vi "DoNewModule.vi"(8 "error in (no error)":errorcluster, 9 "ModuleParams":T1, 10 "Save Folder":path, 11 "Project in":refnum<vi>) -> (0 "error out":errorcluster, 3 "Project out":refnum<vi>)   [LabVIEW 2024, in "AddNewModule.lvlib"]
uses:
  AddNewModule.lvlib
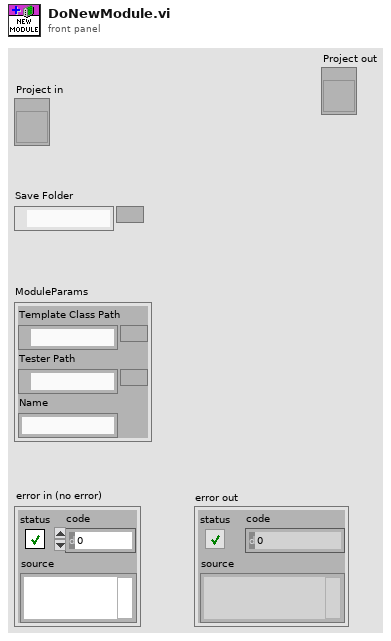
[diagram p1: front panel]
types:
  T1 = cluster{"Template Class Path":path, "Tester Path":path, "Name":string}
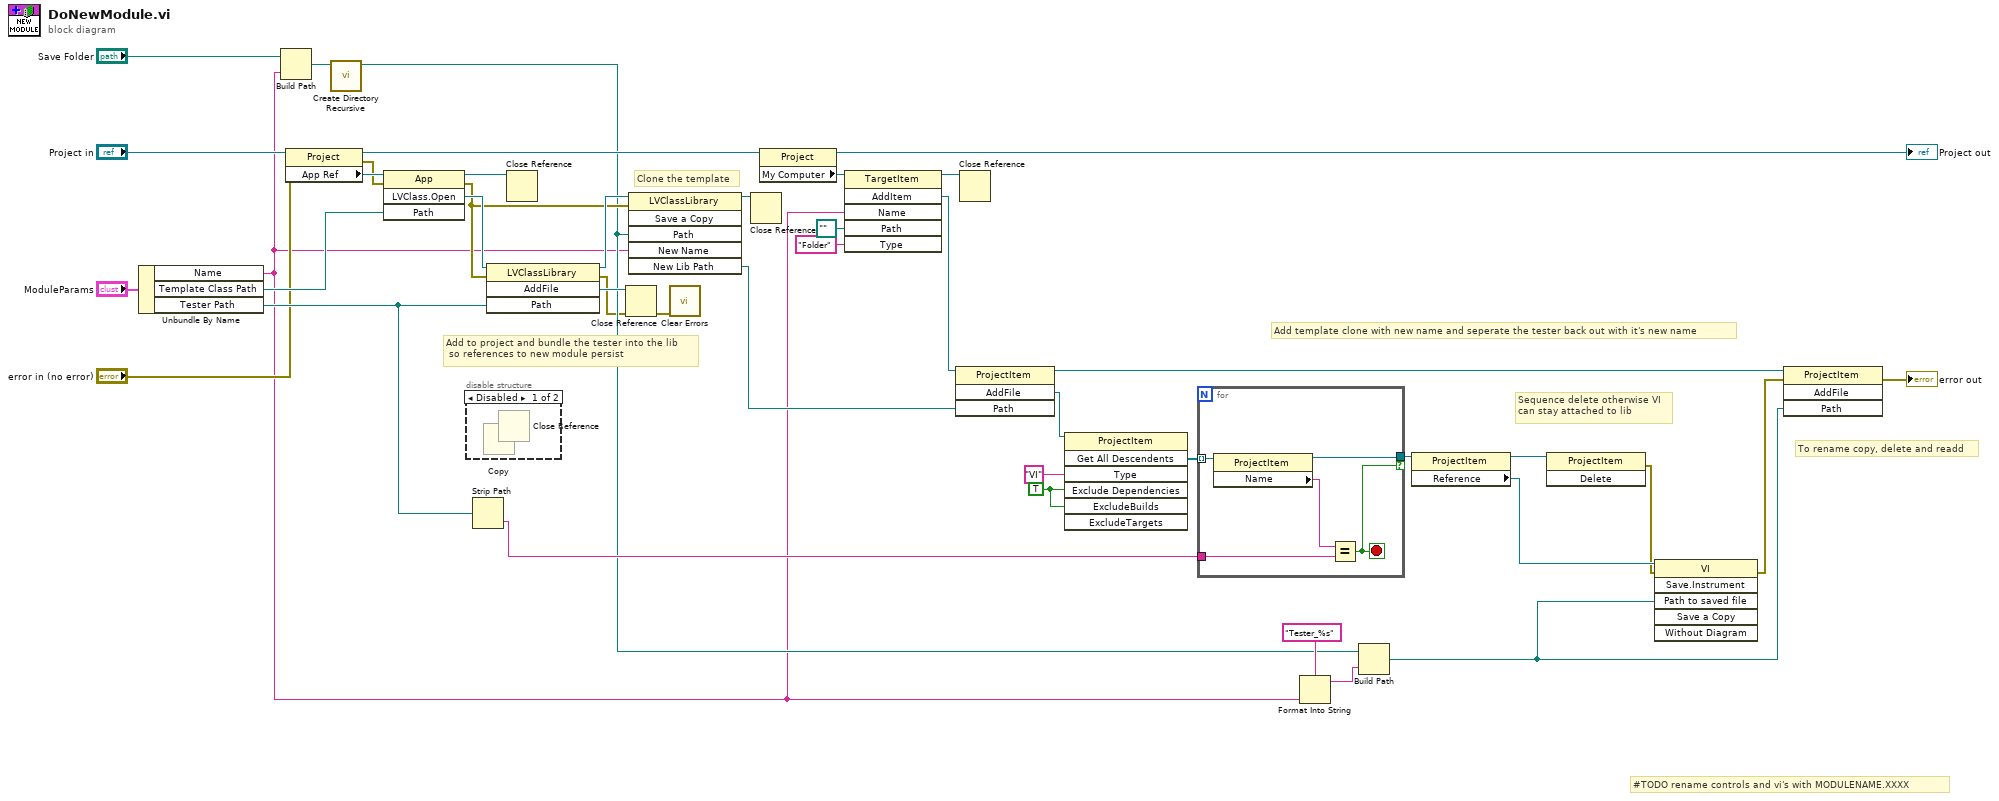
[diagram p0: block diagram]
diagram:
  w21 = TRUE ("ExcludeDependencies")
  # "#TODO rename controls and vi's with MODULENAME.XXXX"
  # "Add template clone with new name and seperate the tester back out with it's new name"
  # "Clone the template"
  # "Add to project and bundle the tester into the lib\n so references to new module persist"
  # "Sequence delete otherwise VI\ncan stay attached to lib"
  # "To rename copy, delete and readd"
  n1 = Unbundle By Name("ModuleParams") -> ("Name"=w1:string, "Template Class Path"=w37:path, "Tester Path"=w24:path)
  n2 = Build Path(base path="Save Folder", name or relative path=w1) -> (appended path=w40:path)
  n3 = property class="Project"(reference="Project in", error in="error in (no error)") -> (reference out=w34:refnum<vi>, error out=w2:errorcluster, "App Ref"=w38:refnum<vi>)
  n4 = call <vilib>:"Create Directory Recursive.vi"("directory"=w40) -> ("directory copy"=w9:path)  [unwired: 4 in, 2 out]
  n5 = invoke class="App" method="LVClass.Open"(reference=w38, error in=w2, "Path"=w37) -> (reference out=w33:refnum<vi>, error out=w30:errorcluster, "LVClass.Open"=w36:refnum<vi>)  [unwired: 1 in, 1 out]
  n6 = disable-structure shown="Disabled" {
    frame Disabled {
      n7 = Copy() -> ()  [unwired: 5 in, 3 out]
      n8 = Close Reference() -> ()  [unwired: 2 in, 1 out]
    }
    frame Enabled {
    }
  }
  n9 = Strip Path(path=w24) -> (name=w14:string)  [unwired: 1 out]
  n10 = invoke class="LVClassLibrary" method="AddFile"(reference=w36, error in=w30, "Path"=w24) -> (reference out=w35:refnum<vi>, error out=w6:errorcluster, "AddFile"=w31:refnum<vi>)  [unwired: 1 in, 1 out]
  n11 = Close Reference(reference=w33) -> ()  [unwired: 1 in, 1 out]
  n12 = Close Reference(reference=w31, error in (no error)=w6) -> (error out=w5:errorcluster)
  n13 = invoke class="LVClassLibrary" method="Save a Copy"(reference=w35, error in=w30, "Path"=w9, "New Name"=w1) -> (reference out=w32:refnum<vi>, "New Lib Path"=w17:path)  [unwired: 2 in, 4 out]
  n14 = call <vilib>:"Clear Errors.vi"("error in (no error)"=w5) -> ()  [unwired: 5 in, 2 out]
  n15 = Close Reference(reference=w32) -> ()  [unwired: 1 in, 1 out]
  n16 = property class="Project"(reference=w34) -> (reference out=→"Project out":refnum<vi>, "My Computer"=w28:refnum<vi>)  [unwired: 1 in, 1 out]
  n17 = invoke class="TargetItem" method="AddItem"(reference=w28, "Name"=w1, "Path"=path "", "Type"="Folder") -> (reference out=w27:refnum<vi>, "AddItem"=w26:refnum<vi>)  [unwired: 2 in, 4 out]
  n18 = invoke class="ProjectItem" method="AddFile"(reference=w26, "Path"=w17) -> (reference out=w10:refnum<vi>, "AddFile"=w23:refnum<vi>)  [unwired: 2 in, 2 out]
  n19 = Close Reference(reference=w27) -> ()  [unwired: 1 in, 1 out]
  n20 = invoke class="ProjectItem" method="Get All Descendents"(reference=w23, "Type"="VI", "Exclude Dependencies"=w21, "ExcludeBuilds"=w21) -> ("All Descendents"=w20:refnum<vi>[])  [unwired: 3 in, 6 out]
  n21 = for {
    tunnel: w20 -> [w47] mode=indexing
    tunnel: w14 -> [w46]
    tunnel: [w44] -> w19 if=w43
    stop <- w43 stop-if-true
    n22 = property class="ProjectItem"(reference=w47) -> (reference out=w44:refnum<vi>, "Name"=w45:string)  [unwired: 1 in, 1 out]
    n23 = Equal?(x=w45, y=w46) -> (x = y?=w43:bool)
  }
  n24 = Format Into String(format string="Tester_%s", w1) -> (resulting string=w16:string)  [unwired: 2 in, 1 out]
  n25 = Build Path(base path=w9, name or relative path=w16) -> (appended path=w12:path)
  n26 = property class="ProjectItem"(reference=w19) -> (reference out=w13:refnum<vi>, "Reference"=w18:refnum<vi>)  [unwired: 1 in, 1 out]
  n27 = invoke class="ProjectItem" method="Delete"(reference=w13) -> (error out=w7:errorcluster)  [unwired: 2 in, 2 out]
  n28 = invoke class="VI" method="Save.Instrument"(reference=w18, error in=w7, "Path to saved file"=w12) -> (error out=w11:errorcluster)  [unwired: 3 in, 5 out]
  n29 = invoke class="ProjectItem" method="AddFile"(reference=w10, error in=w11, "Path"=w12) -> (error out=→"error out":errorcluster)  [unwired: 1 in, 3 out]
